vi "DSF.Engine.Interface.Plugin.Write.Response.vi"(6 "overwrite on timeout (T)":bool, 8 "error in (no error)":errorcluster, 9 "timeout in ms (0)":i32, 10 "response":T1, 11 "Plugin Interface in":refnum<class "DSF.Engine.Interface.Plugin.lvclass">) -> (0 "error out":errorcluster, 1 "timed out?":bool, 3 "Plugin Interface out":refnum<class "DSF.Engine.Interface.Plugin.lvclass">)   [LabVIEW 2017, in "DSF.Engine.lvlib" / "DSF.Engine.Interface.Plugin.lvclass"]
uses:
  DSF.Engine.Interface.Plugin.lvclass
  C:/Git/DSF/Source/Engine/Classes/Interface/DSF.Engine.Interface.lvclass
  DSF.Engine.Interface.Plugin.Response Data.ctl
  DSF.Engine.Interface.Plugin.Response.ctl
  DSF.Engine.Interface.Plugin.Response Parameters.ctl
  DSF.Engine.Interface.lvclass/DSF.Engine.Interface.ctl
  DSF.Engine.Interface.RT FIFO.Data.16B.ctl
  DSF.Engine.Interface.RT FIFO.Payload.16B.ctl
  DSF.Engine.Interface.lvclass
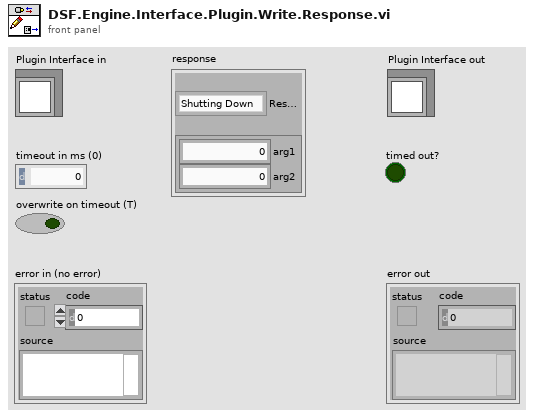
[diagram p1: front panel]
types:
  T1 = typedef "DSF.Engine.lvlib/DSF.Engine.Interface.Plugin.lvclass/DSF.Engine.Interface.Plugin.Response Data.ctl" = cluster{"Response":T2, "Response Parameters":T3}
  T2 = typedef "DSF.Engine.lvlib/DSF.Engine.Interface.Plugin.lvclass/DSF.Engine.Interface.Plugin.Response.ctl" = enum8{"Shutting Down"}
  T3 = typedef "DSF.Engine.lvlib/DSF.Engine.Interface.Plugin.lvclass/DSF.Engine.Interface.Plugin.Response Parameters.ctl" = cluster{"arg1":u64, "arg2":u64}
  T4 = typedef "DSF.Engine.lvlib/DSF.Engine.Interface.lvclass/DSF.Engine.Interface.RT FIFO.Data.16B.ctl" = cluster{"Command":u8, "Payload":T5}
  T5 = typedef "DSF.Engine.lvlib/DSF.Engine.Interface.lvclass/DSF.Engine.Interface.RT FIFO.Payload.16B.ctl" = cluster{"arg1":u64, "arg2":u64}
  T6 = typedef "DSF.Engine.lvlib/DSF.Engine.Interface.lvclass/DSF.Engine.Interface.RT FIFO.Ref.16B.ctl" = refnum<k33>
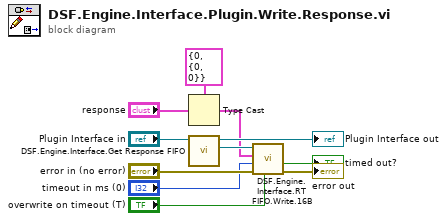
[diagram p0: block diagram]
diagram:
  n1 = Type Cast(type=T4 {"Command"=0, "Payload"={"arg1"=0, "arg2"=0}} ("element"), x="response") -> (*(type *) &x=w3:T4)
  n2 = call "DSF.Engine.Interface.Get Response FIFO.vi"("Interface in"="Plugin Interface in") -> ("Response FIFO"=w9:T6, "Interface out"=→"Plugin Interface out":refnum<class "DSF.Engine.Interface.Plugin.lvclass">)  [unwired: 9 in]
  n3 = call "DSF.Engine.Interface.RT FIFO.Write.16B.vi"("overwrite on timeout (T)"="overwrite on timeout (T)", "error in (no error)"="error in (no error)", "timeout in ms (0)"="timeout in ms (0)", "element"=w3, "RT FIFO in"=w9) -> ("error out"=→"error out":errorcluster, "timed out?"=→"timed out?":bool)  [unwired: 4 in, 1 out]
